vi "Parse-attribute.vi"(8 "error in (no error)":errorcluster, 10 "String in":string, 11 "Boolean in":refnum<class "Boolean.lvclass">) -> (0 "error out":errorcluster, 1 "Valid attribute?":bool, 2 "Remaining string":string, 3 "Boolean out":refnum<class "Boolean.lvclass">)   [LabVIEW 2013, in "HardwareCharacterization.lvlib" / "Boolean.lvclass"]
uses:
  Boolean.lvclass
  Boolean.lvclass/Boolean.ctl
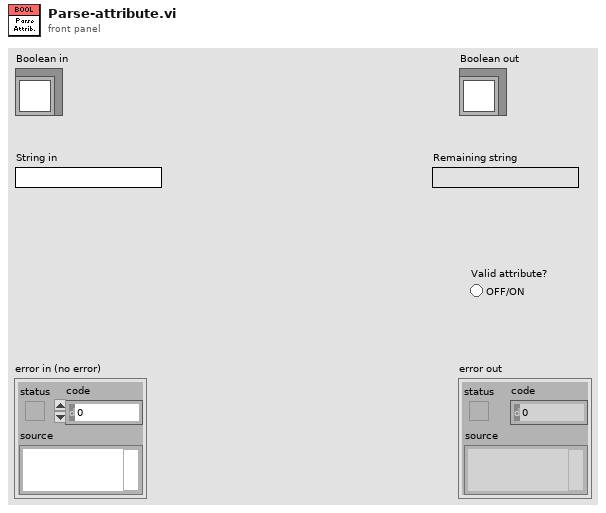
[diagram p1: front panel]
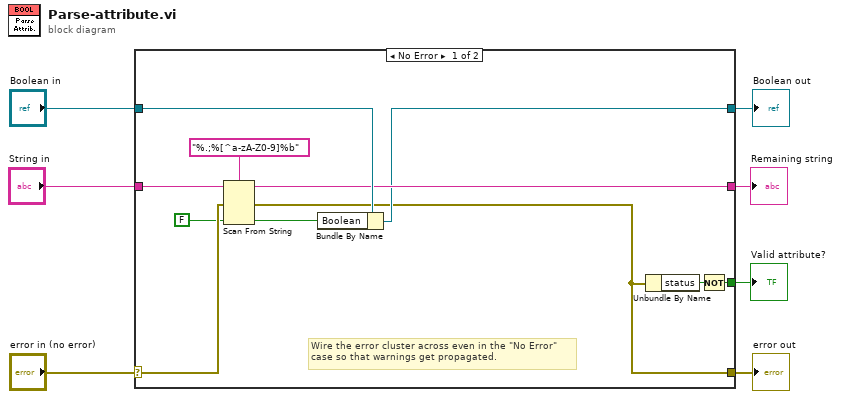
[diagram p0: block diagram]
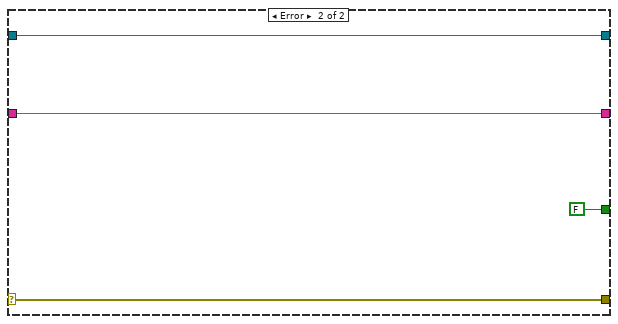
[diagram p2: hidden frame]
diagram:
  n1 = case shown="No Error" "error in (no error)" {
    selector: "error in (no error)" -> [w15 w22]
    tunnel: [w8 w22] -> w6
    tunnel: [w9 w21] -> w4
    tunnel: "Boolean in" -> [w12 w21]
    tunnel: "String in" -> [w16 w20]
    tunnel: [w11 w20] -> w2
    tunnel: [w10 FALSE] -> w1
    frame No Error {
      # "Wire the error cluster across even in the \"No Error\"\ncase so that warnings get propagated."
      n2 = Scan From String(format string="%.;%[^a-zA-Z0-9]%b", input string=w16, error in=w15, default 2=FALSE) -> (remaining string=w11:string, error out=w8:errorcluster, output 2=w13:bool)  [unwired: 3 in, 1 out]
      n3 = Bundle By Name(cluster=w12, "Boolean"=w13) -> (w9:refnum<class "Boolean.lvclass">)
      n4 = Unbundle By Name(w8) -> ("status"=w17:bool)
      n5 = Not(x=w17) -> (.not. x?=w10:bool)
    }
    frame Error {
    }
  }
  "error out" <- w6
  "Boolean out" <- w4
  "Valid attribute?" <- w1
  "Remaining string" <- w2
